vi "authorize.vi"(7 "httpRequestID":u32) -> ()   [LabVIEW 2011]
doc: "This VI is a state machine that can be ran from a Browser."
uses:
  server/database/Users/User Record.ctl
  <vilib>/addons/internet/utils/strutil.llb/Case Matching.ctl
  <vilib>/wsapi/NI_WebServices.lvlib
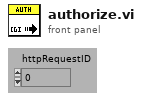
[diagram p1: front panel]
types:
  T1 = typedef "User Record.ctl" = cluster{"ixUser":i32, "sxUsername":string, "sLastName":string, "sFirstName":string, "sEmail":string, "sPassword":string, "tLoginTime":timestamp, "sLoginComputer":string, "fAdministrator":bool, "fRunSequences":bool, "fModifySequences":bool, "fRunScenarios":bool, "fModifyScenarios":bool, "fModifyTemplates":bool, "fModifyUsers":bool, "fModifyStations":bool, "fModifyFields":bool}
  T2 = typedef "Connection Refnum.ctl" = cluster{"Environment Handle":i32, "Connection Handle":i32}
  T3 = typedef "Case Matching.ctl" = enum16{"a != A", "a == A", "system"}
  T4 = typedef "Keyed Array.ctl" = cluster{"keys":string[], "values":string[]}
  T5 = typedef "Authorization Data.ctl" = cluster{"Valid":bool, "Seats":i32, "Expire Time":timestamp, "Last Access Time":timestamp, "Product ID":string, "Hardware ID":string, "Spartan Serial Number":string, "Feature":cluster{"#attributes":cluster{"Name":string, "Value":string}}[]}
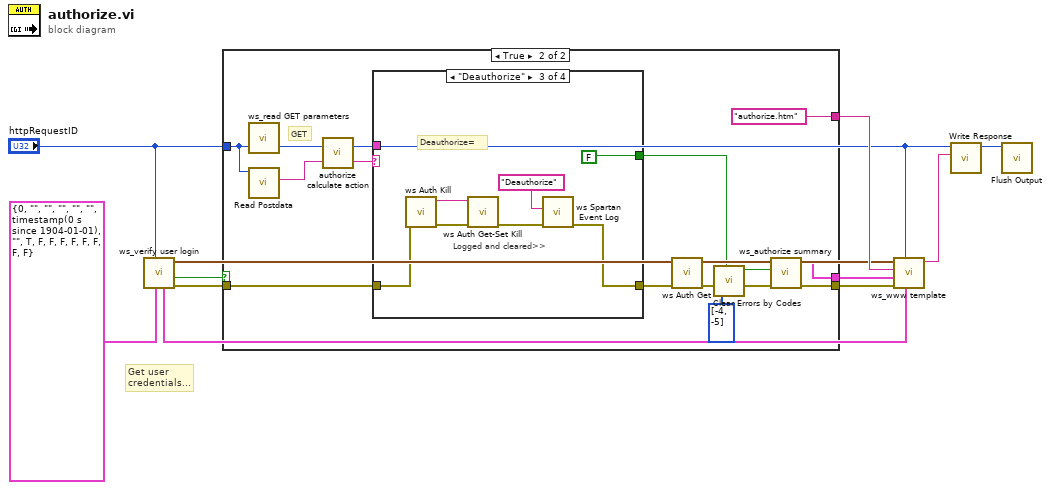
[diagram p0: block diagram]
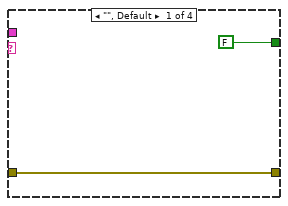
[diagram p3: hidden frame]
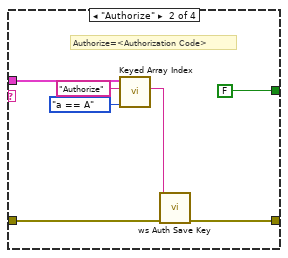
[diagram p4: hidden frame]
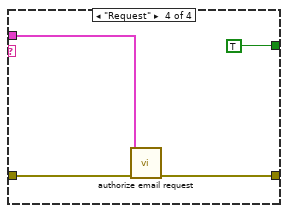
[diagram p5: hidden frame]
diagram:
  # "Get user \ncredentials..."
  n1 = call "ws_verify user login.vi"("Required Permisions"=T1 {"ixUser"=0, "sxUsername"="", "sLastName"="", "sFirstName"="", "sEmail"="", "sPassword"="", "tLoginTime"=timestamp(0 s since 1904-01-01), "sLoginComputer"="", "fAdministrator"=TRUE, "fRunSequences"=FALSE, "fModifySequences"=FALSE, "fRunScenarios"=FALSE, "fModifyScenarios"=FALSE, "fModifyTemplates"=FALSE, "fModifyUsers"=FALSE, "fModifyStations"=FALSE, "fModifyFields"=FALSE} ("User Record"), "httpRequestID"="httpRequestID") -> ("error out"=w11:errorcluster, "User Verified\nand Spartan\nAuthorized?"=w10:bool, "DB Connection Ref"=w4:T2, "User"=w7:T1)  [unwired: 6 in]
  n2 = case shown="True" w10 {
    tunnel: w11 -> [w12 w22]
    tunnel: [w12 w17] -> w8
    tunnel: [_ w18] -> w6
    tunnel: [_ "authorize.htm"] -> w5
    tunnel: "httpRequestID" -> [_ w14]
    frame False {
      # "Spartan is not authorized or User does not have permission"
    }
    frame True {
      # "GET"
      n3 = call "ws_read GET parameters.vi"("httpRequestID"=w14) -> ("GET query params"=w15:T4)  [unwired: 2 in]
      n4 = call <vilib>:"Read Postdata.vi"("httpRequestID"=w14) -> ("postdata"=w13:string)  [unwired: 8 in, 2 out]
      n5 = call "authorize calculate action.vi"("Content (\"\")"=w13, "Query Params"=w15) -> ("Action"=w21:string, "Query Params"=w20:T4)
      n6 = case shown="\"Deauthorize\"" w21 {
        tunnel: [w29 w36 w39 w45] -> w23
        tunnel: w22 -> [w29 w35 w38 w46]
        tunnel: w20 -> [_ w33 _ w44]
        tunnel: [FALSE FALSE FALSE TRUE] -> w19
        frame "", Default {
        }
        frame "Authorize" {
          # "Authorize=<Authorization Code>"
          n7 = call <vilib>:"Keyed Array Index.vi"("case matching (sensitive)"=Case_Matching."a == A", "key"="Authorize", "array in"=w33) -> ("value"=w30:string)  [unwired: 1 in, 3 out]
          n8 = call "ws Auth Save Key.vi"("error in (no error)"=w35, "Site Key"=w30) -> ("error out"=w36:errorcluster)  [unwired: 9 in]
        }
        frame "Deauthorize" {
          # "Deauthorize="
          # "Logged and cleared>>"
          n9 = call "ws Auth Kill.vi"("error in (no error)"=w38) -> ("error out"=w40:errorcluster, "Confirm Code"=w41:string)  [unwired: 9 in]
          n10 = call "ws Auth Get-Set Kill.vi"("error in (no error)"=w40, "KillCode to Set (empty - read existing)"=w41) -> ("error out"=w42:errorcluster)  [unwired: 8 in, 1 out]
          n11 = call "ws Spartan Event Log.vi"("error in (no error)"=w42, "module (\"\")"="Deauthorize" ("module (\"\")")) -> ("error out"=w39:errorcluster)  [unwired: 6 in]
        }
        frame "Request" {
          n12 = call "authorize email request.vi"("error in (no error)"=w46, "POST (empty)"=w44) -> ("error out"=w45:errorcluster)  [unwired: 9 out]
        }
      }
      n13 = call "ws Auth Get.vi"("error in (no error)"=w23) -> ("error out"=w26:errorcluster, "Authorization"=w25:T5)  [unwired: 9 in]
      n14 = call "Clear Errors by Codes.vi"("Error Codes\nto Clear (Empty)"=i32[] [-4, -5] ("Error Codes\nto Clear (Empty)"), "error in (no error)"=w26) -> ("error out"=w24:errorcluster)  [unwired: 5 out]
      n15 = call "ws_authorize summary.vi"("error in (no error)"=w24, "Authorization Request Sent? (f)"=w19, "Authorization"=w25) -> ("error out"=w17:errorcluster, "Template Keys"=w18:T4)  [unwired: 3 out]
    }
  }
  n16 = call "ws_www template.vi"("User"=w7, "httpRequestID"="httpRequestID", "error in (no error)"=w8, "Template Keys (empty)"=w6, "Template (\"\")"=w5, "DB Connection Ref"=w4) -> ("HTTP Template Content"=w2:string)  [unwired: 5 in]
  n17 = call <vilib>:"Write Response.vi"("response string"=w2, "httpRequestID"="httpRequestID") -> ("httpRequestID out"=w1:u32)  [unwired: 8 in, 1 out]
  n18 = call <vilib>:"Flush Output.vi"("httpRequestID"=w1) -> ()  [unwired: 9 in, 2 out]
